vi "Get Magnet.vi"(6 "Axis":T1=enum."Z", 8 "error in (no error)":errorcluster, 11 "Instrument.Cryostat in":refnum<class "Instrument.Cryostat.lvclass">) -> (0 "error out":errorcluster, 1 "Status":string, 2 "B Field (T)":dbl, 3 "Instrument.Cryostat out":refnum<class "Instrument.Cryostat.lvclass">, 4 "Finished?":bool)   [LabVIEW 2019, in "Instrument.Cryostat.lvclass"]
uses:
  Instrument.Cryostat.lvclass
  Typedefs/Magnet Axis--Enum.ctl
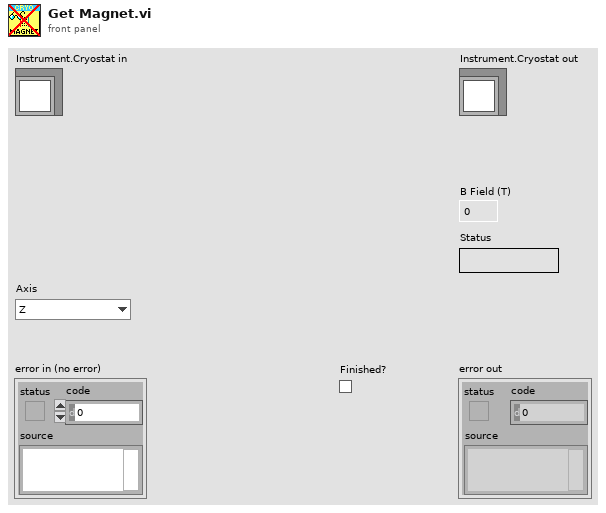
[diagram p1: front panel]
types:
  T1 = typedef "Instrument.Cryostat.lvclass/Magnet Axis--Enum.ctl" = enum16{"X", "Y", "Z"}
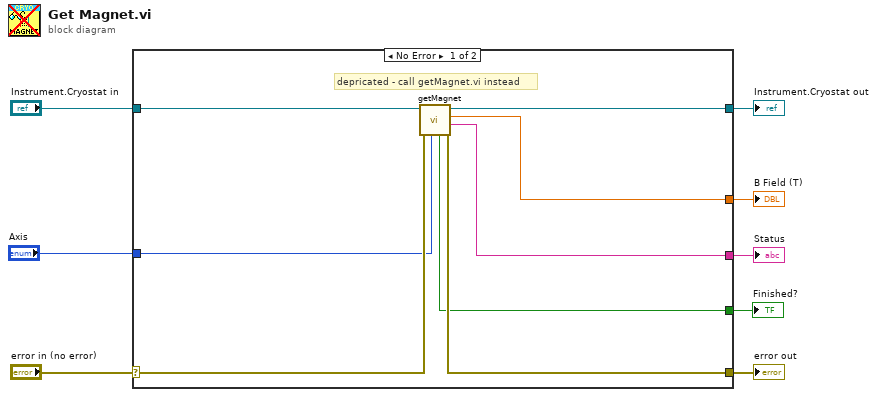
[diagram p0: block diagram]
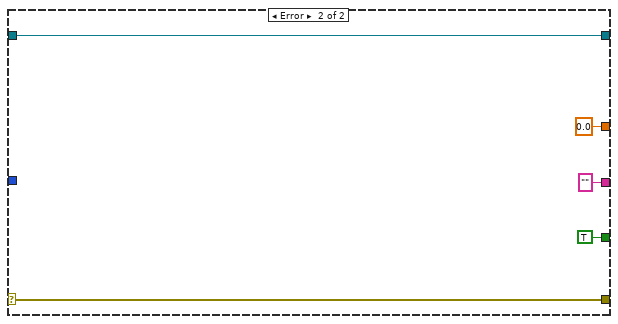
[diagram p2: hidden frame]
diagram:
  n1 = case shown="No Error" "error in (no error)" {
    selector: "error in (no error)" -> [w14 w21]
    tunnel: [w13 w21] -> w7
    tunnel: [w16 w20] -> w5
    tunnel: "Instrument.Cryostat in" -> [w15 w20]
    tunnel: "Axis" -> [w12 _]
    tunnel: [w11 TRUE ("Finished?")] -> w3
    tunnel: [w10 "" ("Status")] -> w2
    tunnel: [w9 0.0 ("B Field (T)")] -> w1
    frame No Error {
      # "depricated - call getMagnet.vi instead"
      n2 = call-dynamic "getMagnet.vi"("Axis"=w12, "error in (no error)"=w14, "Instrument.Cryostat in"=w15) -> ("error out"=w13:errorcluster, "Status"=w10:string, "B Field (T)"=w9:dbl, "Instrument.Cryostat out"=w16:refnum<class "Instrument.Cryostat.lvclass">, "Finished?"=w11:bool)  [unwired: 4 in]
    }
    frame Error {
    }
  }
  "error out" <- w7
  "Instrument.Cryostat out" <- w5
  "B Field (T)" <- w1
  "Status" <- w2
  "Finished?" <- w3
